vi "stepperLeadScrewFGVTest.vi"() -> ()   [LabVIEW 2019]
panel:
  in  "Set LC (cm)":dbl=5.0 format="%#_13g"
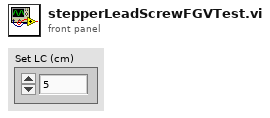
[diagram p1: front panel]
types:
  T1 = typedef "miniRef.ctl" = cluster{"Custom FPGA Reference":refnum<k20>, "error out":errorcluster}
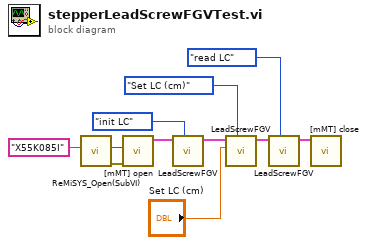
[diagram p0: block diagram]
diagram:
  n1 = call <vilib>:"ReMiSYS_Open(SubVI).vi"("ReMiSYS Key"="X55K085I") -> ("error out"=w11:errorcluster, "Correct Key?"=w10:bool)  [unwired: 9 in]
  n2 = call <vilib>:"[mMT] open.vi"("error in"=w11, "Servo6,7"=w10) -> ("miniOut"=w8:T1)  [unwired: 7 in, 2 out]
  n3 = call "LeadScrewFGV.vi"("Function"=enum16{"init LC", "Set LC (cm)", "read LC"}."init LC", "miniOut in"=w8) -> ("miniOut out"=w6:T1)  [unwired: 7 in, 2 out]
  n4 = call "LeadScrewFGV.vi"("Function"=enum16{"init LC", "Set LC (cm)", "read LC"}."Set LC (cm)", "Set LC (cm)"="Set LC (cm)", "miniOut in"=w6) -> ("miniOut out"=w5:T1)  [unwired: 6 in, 2 out]
  n5 = call "LeadScrewFGV.vi"("Function"=enum16{"init LC", "Set LC (cm)", "read LC"}."read LC", "miniOut in"=w5) -> ("miniOut out"=w4:T1)  [unwired: 7 in, 2 out]
  n6 = call <vilib>:"[mMT] close.vi"("miniOut in"=w4) -> ()  [unwired: 10 in, 1 out]
